vi "FRCts20_Backend_Event_GET.vi"(6 "Message Attributes":T4, 8 "error in (no error)":errorcluster, 10 "Data":string, 11 "Engine_Refnums":T1) -> (0 "error out":errorcluster)   [LabVIEW 2013, in "FRCts20_Backend_Engine.lvlib"]
doc: "Retrieves a specific event's data, called by the Event API. Expects an event index"
uses:
  FRCts20_Backend_Engine.lvlib
  Dependencies/Keyed Array/KeyedArray.ctl
  FRCts20_Backend_EngineRefnums.ctl
  INI_Accessor/FRCts20_Backend_INI Controller.lvclass
  Dependencies/AMC/_SubVIs/TypeDefs/Message Queue.ctl
  Dependencies/AMC/_SubVIs/TypeDefs/Message.ctl
  <vilib>/addons/database/Connection.llb/Conn ObjectReference.ctl
  FRCts20_Backend_API/FRCts20_Backend_API_Event.ctl
  FRCts20_Backend_API/FRCts20_Backend_API_SW.ctl
  FRCts20_Backend_FGVOperation.ctl
  FRCts20_Backend_API/FRCts20_Backend_API.lvlib
  Dependencies/Keyed Array/Tools_KeyedArray.lvlib
  Dependencies/AMC/AMC.lvlib
  <vilib>/addons/database/NI_Database_API.lvlib
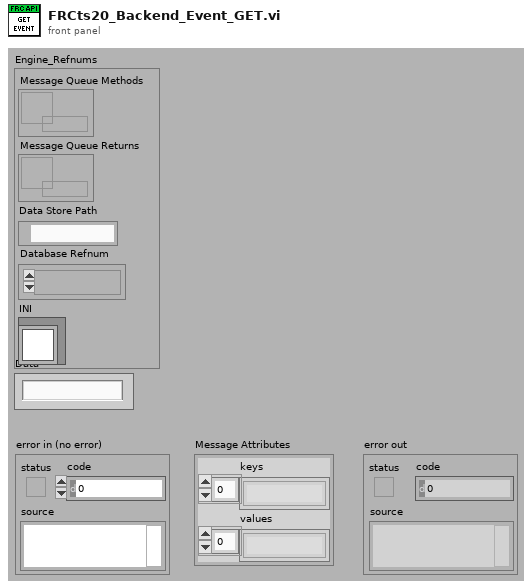
[diagram p1: front panel]
types:
  T1 = typedef "FRCts20_Backend_Engine.lvlib/FRCts20_Backend_EngineRefnums.ctl" = cluster{"Message Queue Methods":T2, "Message Queue Returns":T2, "Data Store Path":path, "Database Refnum":T3, "INI":refnum<class "FRCts20_Backend_INI Controller.lvclass">}
  T2 = typedef "AMC.lvlib/Message Queue.ctl" = refnum<queue>
  T3 = typedef "NI_Database_API.lvlib/Conn ObjectReference.ctl" = refnum<k1>
  T4 = typedef "Tools_KeyedArray.lvlib/KeyedArray.ctl" = cluster{"keys":string[], "values":string[]}
  T5 = typedef "FRCts20_Backend_Engine.lvlib/FRCts20_Backend_FGVOperation.ctl" = enum16{"Initialize", "EnqueueMessage", "EnqueueDataReturn", "FlushMessage", "FlushDataReturn"}
  T6 = typedef "FRCts20_Backend_API.lvlib/FRCts20_Backend_API_Event.ctl" = cluster{"Event Index":u32, "Name":string, "Start Time":timestamp, "End Time":timestamp, "Teams":cluster{"Team Index":u32, "Team Number":u32, "Requests":cluster{"Request Number":u32, "Description":string}[], "Has Open Issue":bool}[], "SWType":T7, "APIReturn":string}
  T7 = typedef "FRCts20_Backend_API.lvlib/FRCts20_Backend_API_SW.ctl" = string
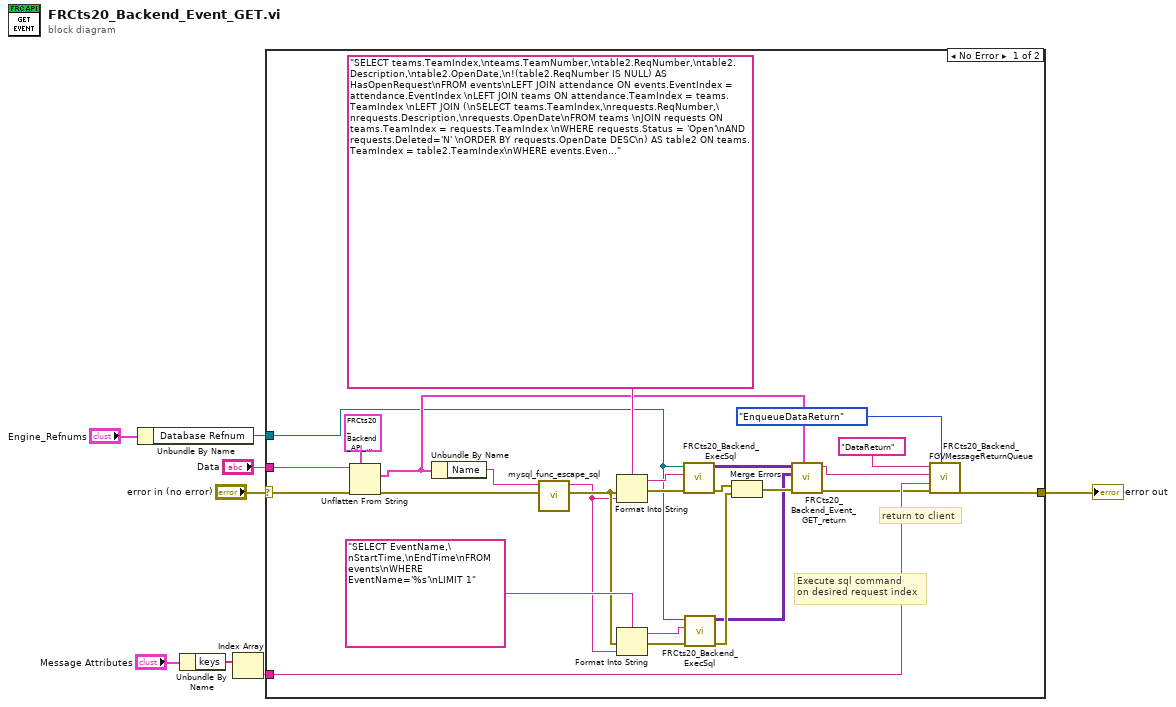
[diagram p0: block diagram]
diagram:
  n1 = Unbundle By Name("Engine_Refnums") -> ("Database Refnum"=w1:T3)
  n2 = Unbundle By Name("Message Attributes") -> ("keys"=w4:string[])
  n3 = Index Array(array=w4) -> (element=w3:string)  [unwired: 1 in]
  n4 = case shown="No Error" "error in (no error)" {
    selector: "error in (no error)" -> [w31 w35]
    tunnel: [w34 w35] -> w7
    tunnel: w1 -> [w18 _]
    tunnel: "Data" -> [w32 _]
    tunnel: w3 -> [w33 _]
    frame No Error {
      # "return to client"
      # "Execute sql command\non desired request index"
      n5 = Unflatten From String(type=T6 {"Event Index"=0, "Name"="", "Start Time"=timestamp(0 s since 1904-01-01), "End Time"=timestamp(0 s since 1904-01-01), "Teams"=[], "SWType"="", "APIReturn"=""} ("Competition"), binary string=w32, error in (no error)=w31) -> (value=w23:T6, error out=w12:errorcluster)  [unwired: 2 in, 1 out]
      n6 = Unbundle By Name(w23) -> ("Name"=w10:string)
      n7 = call "mysql_func_escape_sql.vi"("error in (no error)"=w12, "sqlin"=w10) -> ("error out"=w11:errorcluster, "escaped"=w9:string)  [unwired: 8 in]
      n8 = Format Into String(format string="SELECT teams.TeamIndex,\nteams.TeamNumber,\ntable2.ReqNumber,\ntable2.Description,\ntable2.OpenDate,\n!(table2.ReqNumber IS NULL) AS HasOpenRequest\nFROM events\nLEFT JOIN attendance ON events.EventIndex = attendance.EventIndex \nLEFT JOIN teams ON attendance.TeamIndex = teams.TeamIndex \nLEFT JOIN (\nSELECT teams.TeamIndex,\nrequests.ReqNumber,\nrequests.Description,\nrequests.OpenDate\nFROM teams \nJOIN requests ON teams.TeamIndex = requests.TeamIndex \nWHERE requests.Status = 'Open'\nAND requests.Deleted='N' \nORDER BY requests.OpenDate DESC\n) AS table2 ON teams.TeamIndex = table2.TeamIndex\nWHERE events.EventName='%s'\nORDER BY teamNumber DESC", error in=w11, w9) -> (resulting string=w24:string, error out=w25:errorcluster)  [unwired: 1 in]
      n9 = Format Into String(format string="SELECT EventName,\nStartTime,\nEndTime\nFROM events\nWHERE EventName='%s'\nLIMIT 1", error in=w11, w9) -> (resulting string=w17:string, error out=w19:errorcluster)  [unwired: 1 in]
      n10 = call "FRCts20_Backend_ExecSql.vi"("error in (no error)"=w25, "format string"=w24, "Refnum in"=w18) -> ("error out"=w15:errorcluster, "recordset data"=w21:variant[][])  [unwired: 6 in, 1 out]
      n11 = call "FRCts20_Backend_ExecSql.vi"("error in (no error)"=w19, "format string"=w17, "Refnum in"=w18) -> ("error out"=w14:errorcluster, "recordset data"=w13:variant[][])  [unwired: 6 in, 1 out]
      n12 = Merge Errors(w15, w14) -> (w16:errorcluster)
      n13 = call "FRCts20_Backend_Event_GET_return.vi"("Event"=w23, "error in (no error)"=w16, "recordset data 2"=w13, "recordset data"=w21) -> ("error out"=w27:errorcluster, "data string"=w28:string)  [unwired: 6 in]
      n14 = call "FRCts20_Backend_FGVMessageReturnQueue.vi"("Operation"=FRCts20_Backend_FGVOperation."EnqueueDataReturn", "error in (no error)"=w27, "Key"=w33, "Message Value"=w28, "Message Name"="DataReturn") -> ("error out"=w34:errorcluster)  [unwired: 5 in, 1 out]
    }
    frame Error {
    }
  }
  "error out" <- w7
